vi "Configure Trigger (TV).vi"(0 "VISA resource name":refnum<visa-resource-name>, 1 "TV Trigger Mode (0: All Fields)":i32(ring) items=["All Fields", "All Lines", "Alternate", "Fields1", "Fields2", "Line"], 5 "Trigger Source (1: Channel1)":i32(ring)=1 items=["Channel1"=1, "Channel2"=2, "Channel3"=3, "Channel4"=4], 7 "Horizontal Line Number (1)":i32=1, 9 "Trigger Polarity (0: Negative)":i32(ring) items=["Negative", "Positive"], 11 "error in (no error)":errorcluster, 12 "TV Standard (0: I1080L60HZ)":i32(ring) items=["HDTV (1080i/60)", "HDTV (1080i/50)", "NTSC,PAL-M (525/60)", "PAL,SECAM (625/50)", "EDTV (480p/60)", "EDTV (576p/60)", "HDTV (720p/60)", "HDTV (720p/50)", "HDTV (1080p/60)", "HDTV (1080p/50)", "HDTV (1080p/40)", "HDTV (1080p/30)", "HDTV (1080p/25)", "HDTV (1080p/24)", "User Defined"]) -> (4 "VISA resource name out":refnum<visa-resource-name>, 15 "error out":errorcluster)   [LabVIEW 2013, in "Agilent 90000 Series.lvlib"]
doc: "Configures the TV trigger parameters."
uses:
  Agilent 90000 Series.lvlib
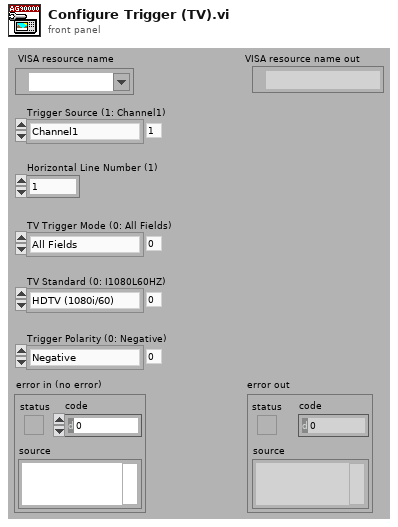
[diagram p1: front panel]
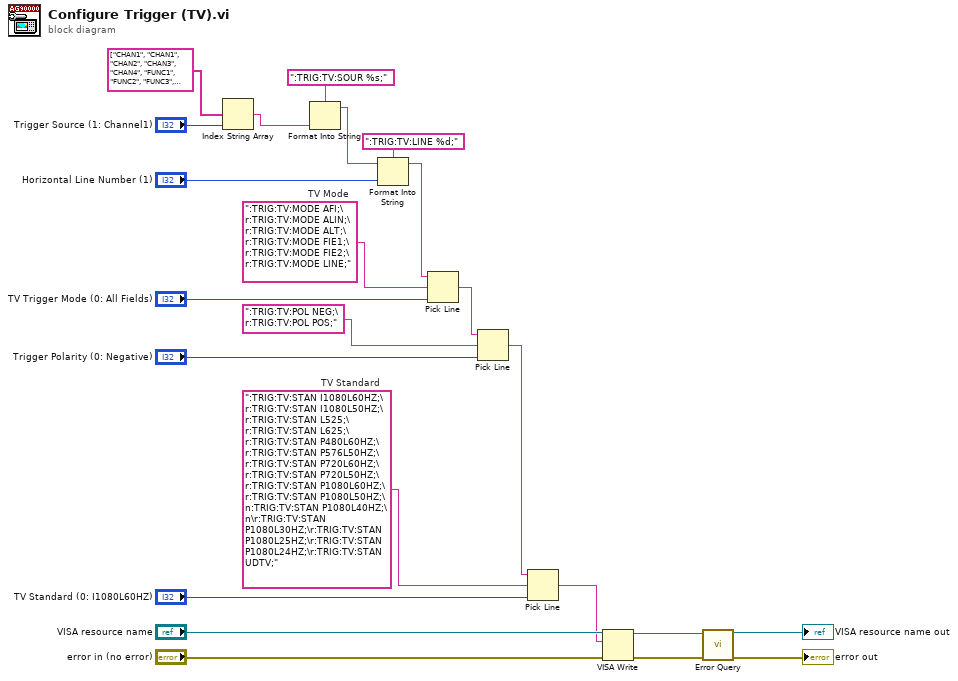
[diagram p0: block diagram]
diagram:
  w15 = ":TRIG:TV:STAN I1080L60HZ;\r:TRIG:TV:STAN I1080L50HZ;\r:TRIG:TV:STAN L525;\r:TRIG:TV:STAN L625;\r:TRIG:TV:STAN P480L60HZ;\r:TRIG:TV:STAN P576L50HZ;\r:TRIG:TV:STAN P720L60HZ;\r:TRIG:TV:STAN P720L50HZ;\r:TRIG:TV:STAN P1080L60HZ;\r:TRIG:TV:STAN P1080L50HZ;\n:TRIG:TV:STAN P1080L40HZ;\n\r:TRIG:TV:STAN P1080L30HZ;\r:TRIG:TV:STAN P1080L25HZ;\r:TRIG:TV:STAN P1080L24HZ;\r:TRIG:TV:STAN UDTV;"  # TV Standard
  w21 = ":TRIG:TV:MODE AFI;\r:TRIG:TV:MODE ALIN;\r:TRIG:TV:MODE ALT;\r:TRIG:TV:MODE FIE1;\r:TRIG:TV:MODE FIE2;\r:TRIG:TV:MODE LINE;"  # TV Mode
  n1 = Index String Array(1:"Trigger Source (1: Channel1)", 2:string[] ["CHAN1", "CHAN1", "CHAN2", "CHAN3", "CHAN4", "FUNC1", "FUNC2", "FUNC3", "FUNC4", "WMEM1", "WMEM2", "WMEM3", "WMEM4", "AUX", "LINE"]) -> (0:w5:string)  [unwired: 1 out]
  n2 = Format Into String(format string=":TRIG:TV:SOUR %s;", w5) -> (resulting string=w3:string)  [unwired: 2 in, 1 out]
  n3 = Format Into String(format string=":TRIG:TV:LINE %d;", initial string=w3, "Horizontal Line Number (1)") -> (resulting string=w2:string)  [unwired: 1 in, 1 out]
  n4 = Pick Line(string ("")=w2, multi-line string=w21, line index="TV Trigger Mode (0: All Fields)") -> (output string=w19:string)
  n5 = Pick Line(string ("")=w19, multi-line string=":TRIG:TV:POL NEG;\r:TRIG:TV:POL POS;", line index="Trigger Polarity (0: Negative)") -> (output string=w16:string)
  n6 = Pick Line(string ("")=w16, multi-line string=w15, line index="TV Standard (0: I1080L60HZ)") -> (output string=w1:string)
  n7 = VISA Write(VISA resource name="VISA resource name", write buffer=w1, error in (no error)="error in (no error)") -> (VISA resource name out=w11:refnum<visa-resource-name>, error out=w10:errorcluster)  [unwired: 1 out]
  n8 = call "Error Query.vi"("error in (no error)"=w10, "VISA resource name"=w11) -> ("error out"=→"error out":errorcluster, "VISA resource name out"=→"VISA resource name out":refnum<visa-resource-name>)  [unwired: 8 out]
